vi "Unsubscribe JSON.vi"(7 "Options":string, 8 "error in (no error)":errorcluster, 9 "Time out ms (1000)":i32=1000, 10 "Topic":string, 11 "WAMP Client in":refnum<class "WAMP Client.lvclass">) -> (0 "error out":errorcluster, 3 "WAMP Client out":refnum<class "WAMP Client.lvclass">)   [LabVIEW 2020, in "wamplv.lvlib" / "WAMP Client.lvclass"]
uses:
  WAMP Client.lvclass
  WAMP Client.lvclass/WAMP Client.ctl
  51763aff-f531-435e-9d49-62bb0d2b803c.vi
  Private/Message loop classes/Subscription details/SubscriptionDetailsParent/SubscriptionDetailsParent.lvclass
  Private/Message loop classes/ErrorOrSuccess JSON/ErrorOrSuccess JSON.lvclass
  C:/local/wamplv/Private/Message loop classes/ErrorOrSuccess/ErrorOrSuccess.lvclass
  C:/local/wamplv/Private/Message loop classes/ErrorOrSuccess JSON/ErrorOrSuccess JSON.lvclass
  TypeDefs/Error or abort detail (JSON).ctl
  wamplv.lvlib
panel:
  out "WAMP Error":T1={"Error URI"="", "Error Arguments"="", "Error ArgumentKw"="{}", "Error Details"="{}", "Associated LabVIEW Error"={"status"=FALSE, "code"=0, "source"=""}}
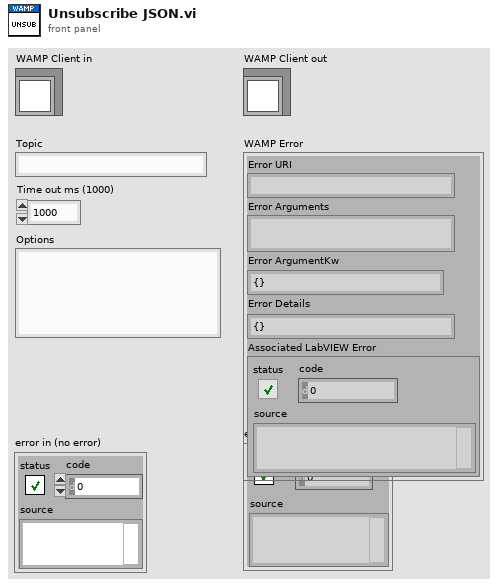
[diagram p1: front panel]
types:
  T1 = typedef "wamplv.lvlib/Error or abort detail (JSON).ctl" = cluster{"Error URI":string, "Error Arguments":string, "Error ArgumentKw":string, "Error Details":string, "Associated LabVIEW Error":errorcluster}
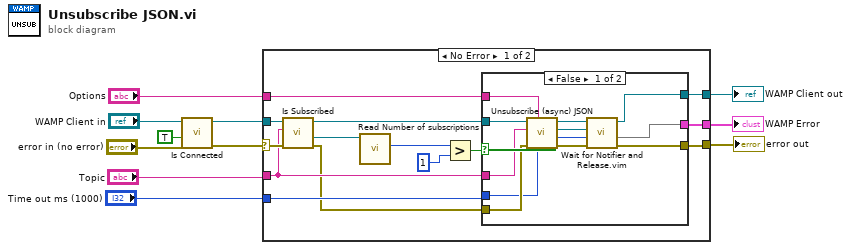
[diagram p0: block diagram]
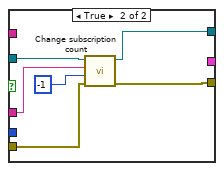
[diagram p2: hidden frame]
diagram:
  n1 = call "Is Connected.vi"("error in"="error in (no error)", "Raise error if not connected"=TRUE, "WAMP Client in"="WAMP Client in") -> ("error out"=w4:errorcluster, "WAMP Client out"=w3:refnum<class "WAMP Client.lvclass">)  [unwired: 6 in, 1 out]
  n2 = case shown="No Error" w4 {
    selector: w4 -> [w19 w44]
    tunnel: [w25 w44] -> w11
    tunnel: [w23 w43] -> w10
    tunnel: w3 -> [w20 w43]
    tunnel: "Time out ms (1000)" -> [w22 _]
    tunnel: "Topic" -> [w18 _]
    tunnel: [w24 _] -> w8
    tunnel: "Options" -> [w21 _]
    frame No Error {
      n3 = call-dynamic "Is Subscribed.vi"("error in (no error)"=w19, "Topic"=w18, "WAMP Client in"=w20) -> ("error out"=w14:errorcluster, "SubscriptionDetailsParent out"=w13:refnum<class "SubscriptionDetailsParent.lvclass">, "WAMP Client out"=w15:refnum<class "WAMP Client.lvclass">)  [unwired: 5 in, 1 out]
      n4 = call "Read Number of subscriptions.vi"("SubscriptionDetailsParent in"=w13) -> ("Number of subscriptions"=w12:u64)  [unwired: 8 in, 2 out]
      n5 = Greater?(x=w12, y=u64 1) -> (0:w16:bool)
      n6 = case shown="False" w16 {
        tunnel: [w36 w39] -> w25
        tunnel: [w30 _] -> w24
        tunnel: [w35 w38] -> w23
        tunnel: w22 -> [w27 _]
        tunnel: w21 -> [w34 _]
        tunnel: w18 -> [w33 w41]
        tunnel: w15 -> [w32 w42]
        tunnel: w14 -> [w31 w37]
        frame False {
          n7 = call-dynamic "Unsubscribe (async) JSON.vi"("Options"=w34, "error in (no error)"=w31, "Topic"=w33, "WAMP Client in"=w32) -> ("error out"=w28:errorcluster, "notifier out"=w26:refnum<notifier>, "WAMP Client out"=w29:refnum<class "WAMP Client.lvclass">)  [unwired: 5 in]
          n8 = call "Wait for Notifier and Release.vim"("error in (no error)"=w28, "timeout in ms (0)"=w27, "Notifier in"=w26, "WAMP Client in"=w29) -> ("error out"=w36:errorcluster, 1:w30, "WAMP Client out"=w35:refnum<class "WAMP Client.lvclass">)  [unwired: 4 in, 1 out]
        }
        frame True {
          n9 = call-dynamic "Change subscription count.vi"("error in (no error)"=w37, "Count change"=i64 -1, "Topic"=w41, "WAMP Client in"=w42) -> ("error out"=w39:errorcluster, "WAMP Client out"=w38:refnum<class "WAMP Client.lvclass">)  [unwired: 6 in]
        }
      }
    }
    frame Error {
    }
  }
  "error out" <- w11
  "WAMP Client out" <- w10
  "WAMP Error" <- w8
